vi "LogError.vi"(8 "entrée d'erreur":errorcluster, 9 "Code":i32, 10 "Source":string, 11 "Error log refnum In":refnum<file>) -> (0 "error out":errorcluster, 3 "Error log refnum out":refnum<file>)   [LabVIEW 2017, in "Logging.lvlib"]
doc: "Ce VI enregistre dans un fichier les messages d'erreur avec leurs définitions et leurs codes.\nEntrée : \nError log refnum In : Refnum du fichier log\nSource : descriptif de l'erreur\ncode : numéro de code de l'erreur (Cf constructeur de l'appareil générant l'erreur)"
uses:
  Logging.lvlib
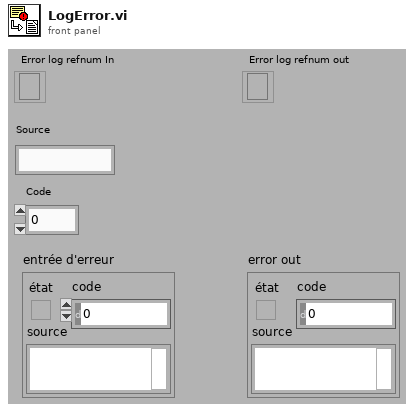
[diagram p1: front panel]
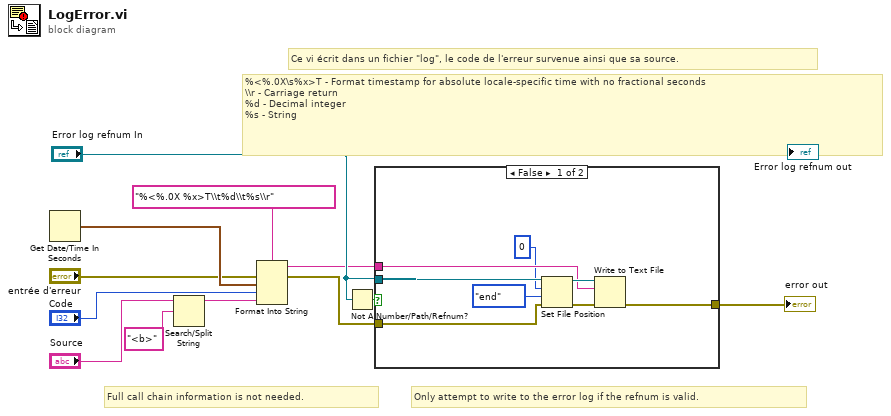
[diagram p0: block diagram]
diagram:
  # "Only attempt to write to the error log if the refnum is valid."
  # "Full call chain information is not needed."
  # "%<%.0X\\s%x>T - Format timestamp for absolute locale-specific time with no fractional seconds\n\\\\r - Carriage return\n%d - Decimal integer\n%s - String"
  # "Ce vi écrit dans un fichier \"log\", le code de l'erreur survenue ainsi que sa source."
  n1 = Get Date/Time In Seconds() -> (seconds since 1Jan1904=w12:timestamp)
  n2 = Search/Split String(string="Source", search string/char (-)="<b>" ("chaîne/car. recherché (-)")) -> (substring before match=w7:string)  [unwired: 1 in, 2 out]
  n3 = Format Into String(format string="%<%.0X %x>T\\t%d\\t%s\\r" ("chaîne de format"), error in="entrée d'erreur", w12, "Code", w7) -> (resulting string=w3:string, error out=w2:errorcluster)  [unwired: 1 in]
  n4 = Not A Number/Path/Refnum?(number/path/refnum="Error log refnum In") -> (NaN/Path/Refnum?=w5:bool)
  n5 = case shown="False" w5 {
    tunnel: "Error log refnum In" -> [w19 _]
    tunnel: w3 -> [w17 _]
    tunnel: w2 -> [w15 w21]
    tunnel: [w13 w21] -> w1
    frame False {
      n6 = Set File Position(offset (in bytes) (0)=i64 0 ("offset (en octets) (0)"), refnum=w19, from (0:start)=enum16{"start", "end", "current"}."end" ("à partir de (0 : start)"), error in=w15) -> (refnum out=w18:refnum<file>, error out=w14:errorcluster)
      n7 = Write to Text File(file (use dialog)=w18, text=w17, error in=w14) -> (error out=w13:errorcluster)  [unwired: 1 in, 2 out]
    }
    frame True {
    }
  }
  "error out" <- w1
  "Error log refnum out" <- "Error log refnum In"
